vi "test Write and Read Signed Integer Array.vi"(8 "error in (no error)":errorcluster, 11 "TestCase in":refnum<class "Read Value Tests.lvclass">) -> (0 "error out":errorcluster, 3 "TestCase out":refnum<class "Read Value Tests.lvclass">)   [LabVIEW 2020, in "Memory Manager Tests.lvlib" / "Read Value Tests.lvclass"]
uses:
  Read Value Tests.lvclass
  Read Value Tests.lvclass/Read Value Tests.ctl
  C:/Program Files/National Instruments/LabVIEW 2027/vi.lib/addons/_JKI Toolkits/VI Tester/TestCase.llb/TestCase.lvclass
  <vilib>/addons/_JKI Toolkits/VI Tester/TestCase.llb/TestCase.lvclass
  Classes/Pointer/Pointer.lvclass
  Classes/Pointer/Read 1D I8.vi
  Classes/Pointer/Read 1D I16.vi
  Classes/Pointer/Read 1D I32.vi
  Classes/Pointer/Read 1D I64.vi
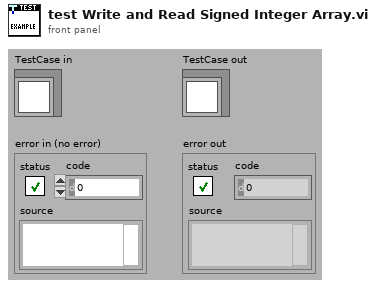
[diagram p1: front panel]
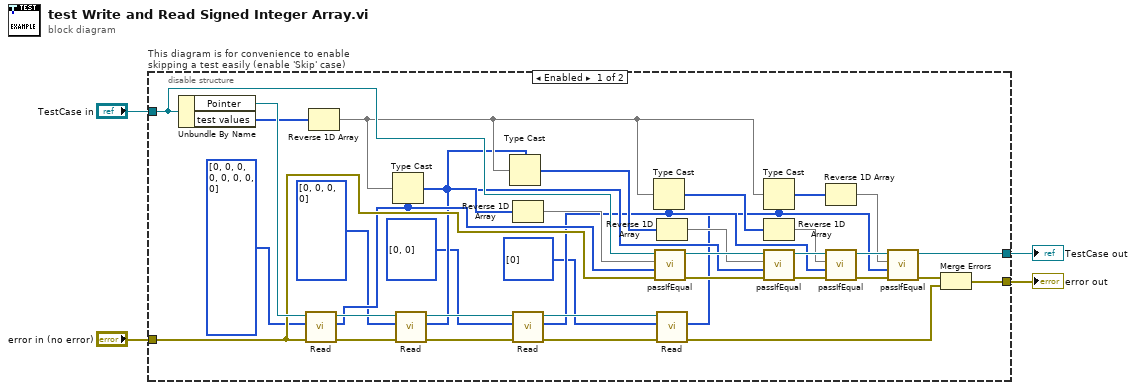
[diagram p0: block diagram]
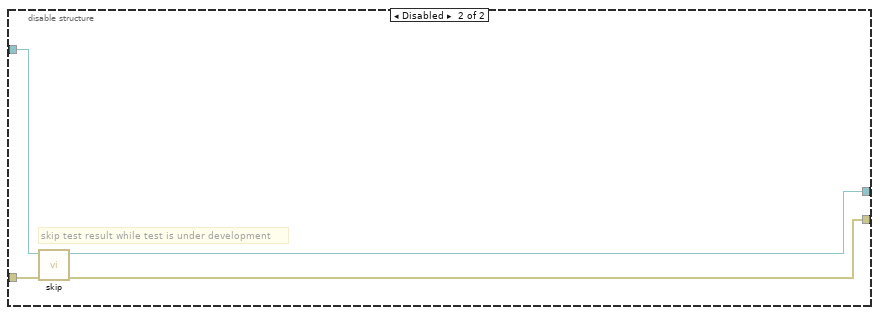
[diagram p2: hidden frame]
diagram:
  n1 = disable-structure "This diagram is for convenience to enable skipping a test easily (enable 'Skip' case)" shown="Enabled" {
    disable-tunnel: "TestCase in" -> [w23 w45]
    disable-tunnel: [w24 w43] -> w1
    disable-tunnel: [w20 w44] -> w3
    disable-tunnel: "error in (no error)" -> [w21 w42]
    frame Enabled {
      n2 = Unbundle By Name(w23) -> ("Pointer"=w22:refnum<class "Pointer.lvclass">, "test values"=w18:u8[])
      n3 = call-poly "Read.vi"("error in (no error)"=w21, "buffer in"=i8[] [0, 0, 0, 0, 0, 0, 0, 0], "Pointer in"=w22) -> ("error out"=w40:errorcluster, "buffer out"=w11:i8[], "Pointer out"=w41:refnum<class "Pointer.lvclass">)  [unwired: 5 in, 1 out]
      n4 = Reverse 1D Array(array=w18) -> (reversed array=w17:u8[])
      n5 = Type Cast(type=w11, x=w17) -> (*(type *) &x=w35:i8[])
      n6 = call-poly "Read.vi"("error in (no error)"=w40, "buffer in"=i16[] [0, 0, 0, 0], "Pointer in"=w41) -> ("error out"=w38:errorcluster, "buffer out"=w9:i16[], "Pointer out"=w39:refnum<class "Pointer.lvclass">)  [unwired: 5 in, 1 out]
      n7 = Type Cast(type=w9, x=w17) -> (*(type *) &x=w34:i16[])
      n8 = Reverse 1D Array(array=w35) -> (reversed array=w16:i8[])
      n9 = call-poly "Read.vi"("error in (no error)"=w38, "buffer in"=i32[] [0, 0], "Pointer in"=w39) -> ("error out"=w36:errorcluster, "buffer out"=w7:i32[], "Pointer out"=w37:refnum<class "Pointer.lvclass">)  [unwired: 5 in, 1 out]
      n10 = Type Cast(type=w7, x=w17) -> (*(type *) &x=w33:i32[])
      n11 = call-dynamic "passIfEqual.vi"("error in (no error)"=w21, "y"=w11, "x"=w16, "TestCase in"=w23) -> ("error out"=w28:errorcluster, "TestCase out"=w29:refnum<class "Read Value Tests.lvclass">)  [unwired: 6 in]
      n12 = Reverse 1D Array(array=w34) -> (reversed array=w15:i16[])
      n13 = call-poly "Read.vi"("error in (no error)"=w36, "buffer in"=i64[] [0], "Pointer in"=w37) -> ("error out"=w19:errorcluster, "buffer out"=w5:i64[])  [unwired: 5 in, 2 out]
      n14 = Type Cast(type=w5, x=w17) -> (*(type *) &x=w32:i64[])
      n15 = Reverse 1D Array(array=w33) -> (reversed array=w14:i32[])
      n16 = call-dynamic "passIfEqual.vi"("error in (no error)"=w28, "y"=w9, "x"=w15, "TestCase in"=w29) -> ("error out"=w26:errorcluster, "TestCase out"=w27:refnum<class "Read Value Tests.lvclass">)  [unwired: 6 in]
      n17 = Reverse 1D Array(array=w32) -> (reversed array=w13:i64[])
      n18 = call-dynamic "passIfEqual.vi"("error in (no error)"=w26, "y"=w7, "x"=w14, "TestCase in"=w27) -> ("error out"=w31:errorcluster, "TestCase out"=w30:refnum<class "Read Value Tests.lvclass">)  [unwired: 6 in]
      n19 = call-dynamic "passIfEqual.vi"("error in (no error)"=w31, "y"=w5, "x"=w13, "TestCase in"=w30) -> ("error out"=w25:errorcluster, "TestCase out"=w24:refnum<class "Read Value Tests.lvclass">)  [unwired: 6 in]
      n20 = Merge Errors(w25, w19) -> (w20:errorcluster)
    }
    frame Disabled {
      # "skip test result while test is under development"
      n21 = call <vilib>:"skip.vi"("error in (no error)"=w42, "TestCase in"=w45) -> ("error out"=w44:errorcluster, "TestCase out"=w43:refnum<class "Read Value Tests.lvclass">)  [unwired: 8 in]
    }
  }
  "error out" <- w3
  "TestCase out" <- w1
